vi "Refrigeration #2.vi"() -> ()   [LabVIEW 2017]
uses:
  Halt Refrig.vi
panel:
  out "Electric Motor Power":dbl caption="W" format="%.1f"
  out "Compressure Suction Pressure":dbl(knob)
  out "Compressor Discharge Pressure":dbl(knob) scale=0.0..60.0
  out "P2":dbl caption="psig" format="%.1g"
  out "P1":dbl caption="psig" format="%.1g"
  out "Evaporator Exit Temperature":dbl format="%.1g"
  out "Evaporator Entrance Temperature":dbl format="%.1g"
  out "Condensor Entrance Temperature":dbl format="%.1g"
  out "Condensor Exit Temperature":dbl format="%.1g"
  out "Compressor Exit Temperature":dbl format="%.1g"
  out "Compressor Entrance Temperature":dbl format="%.1g"
  out "Low Pressure Reciever Temperature":dbl format="%.1g"
  in  "stop":bool
  out "Data Point Count":i32
  in  "Specify Time between Data Points (sec)":dbl=1.0
  in  "Cancel Data Collection":bool
  in  "Specify number of data points":i16=1
  in  "Enable 3":bool
  out "Saving Data 3":bool
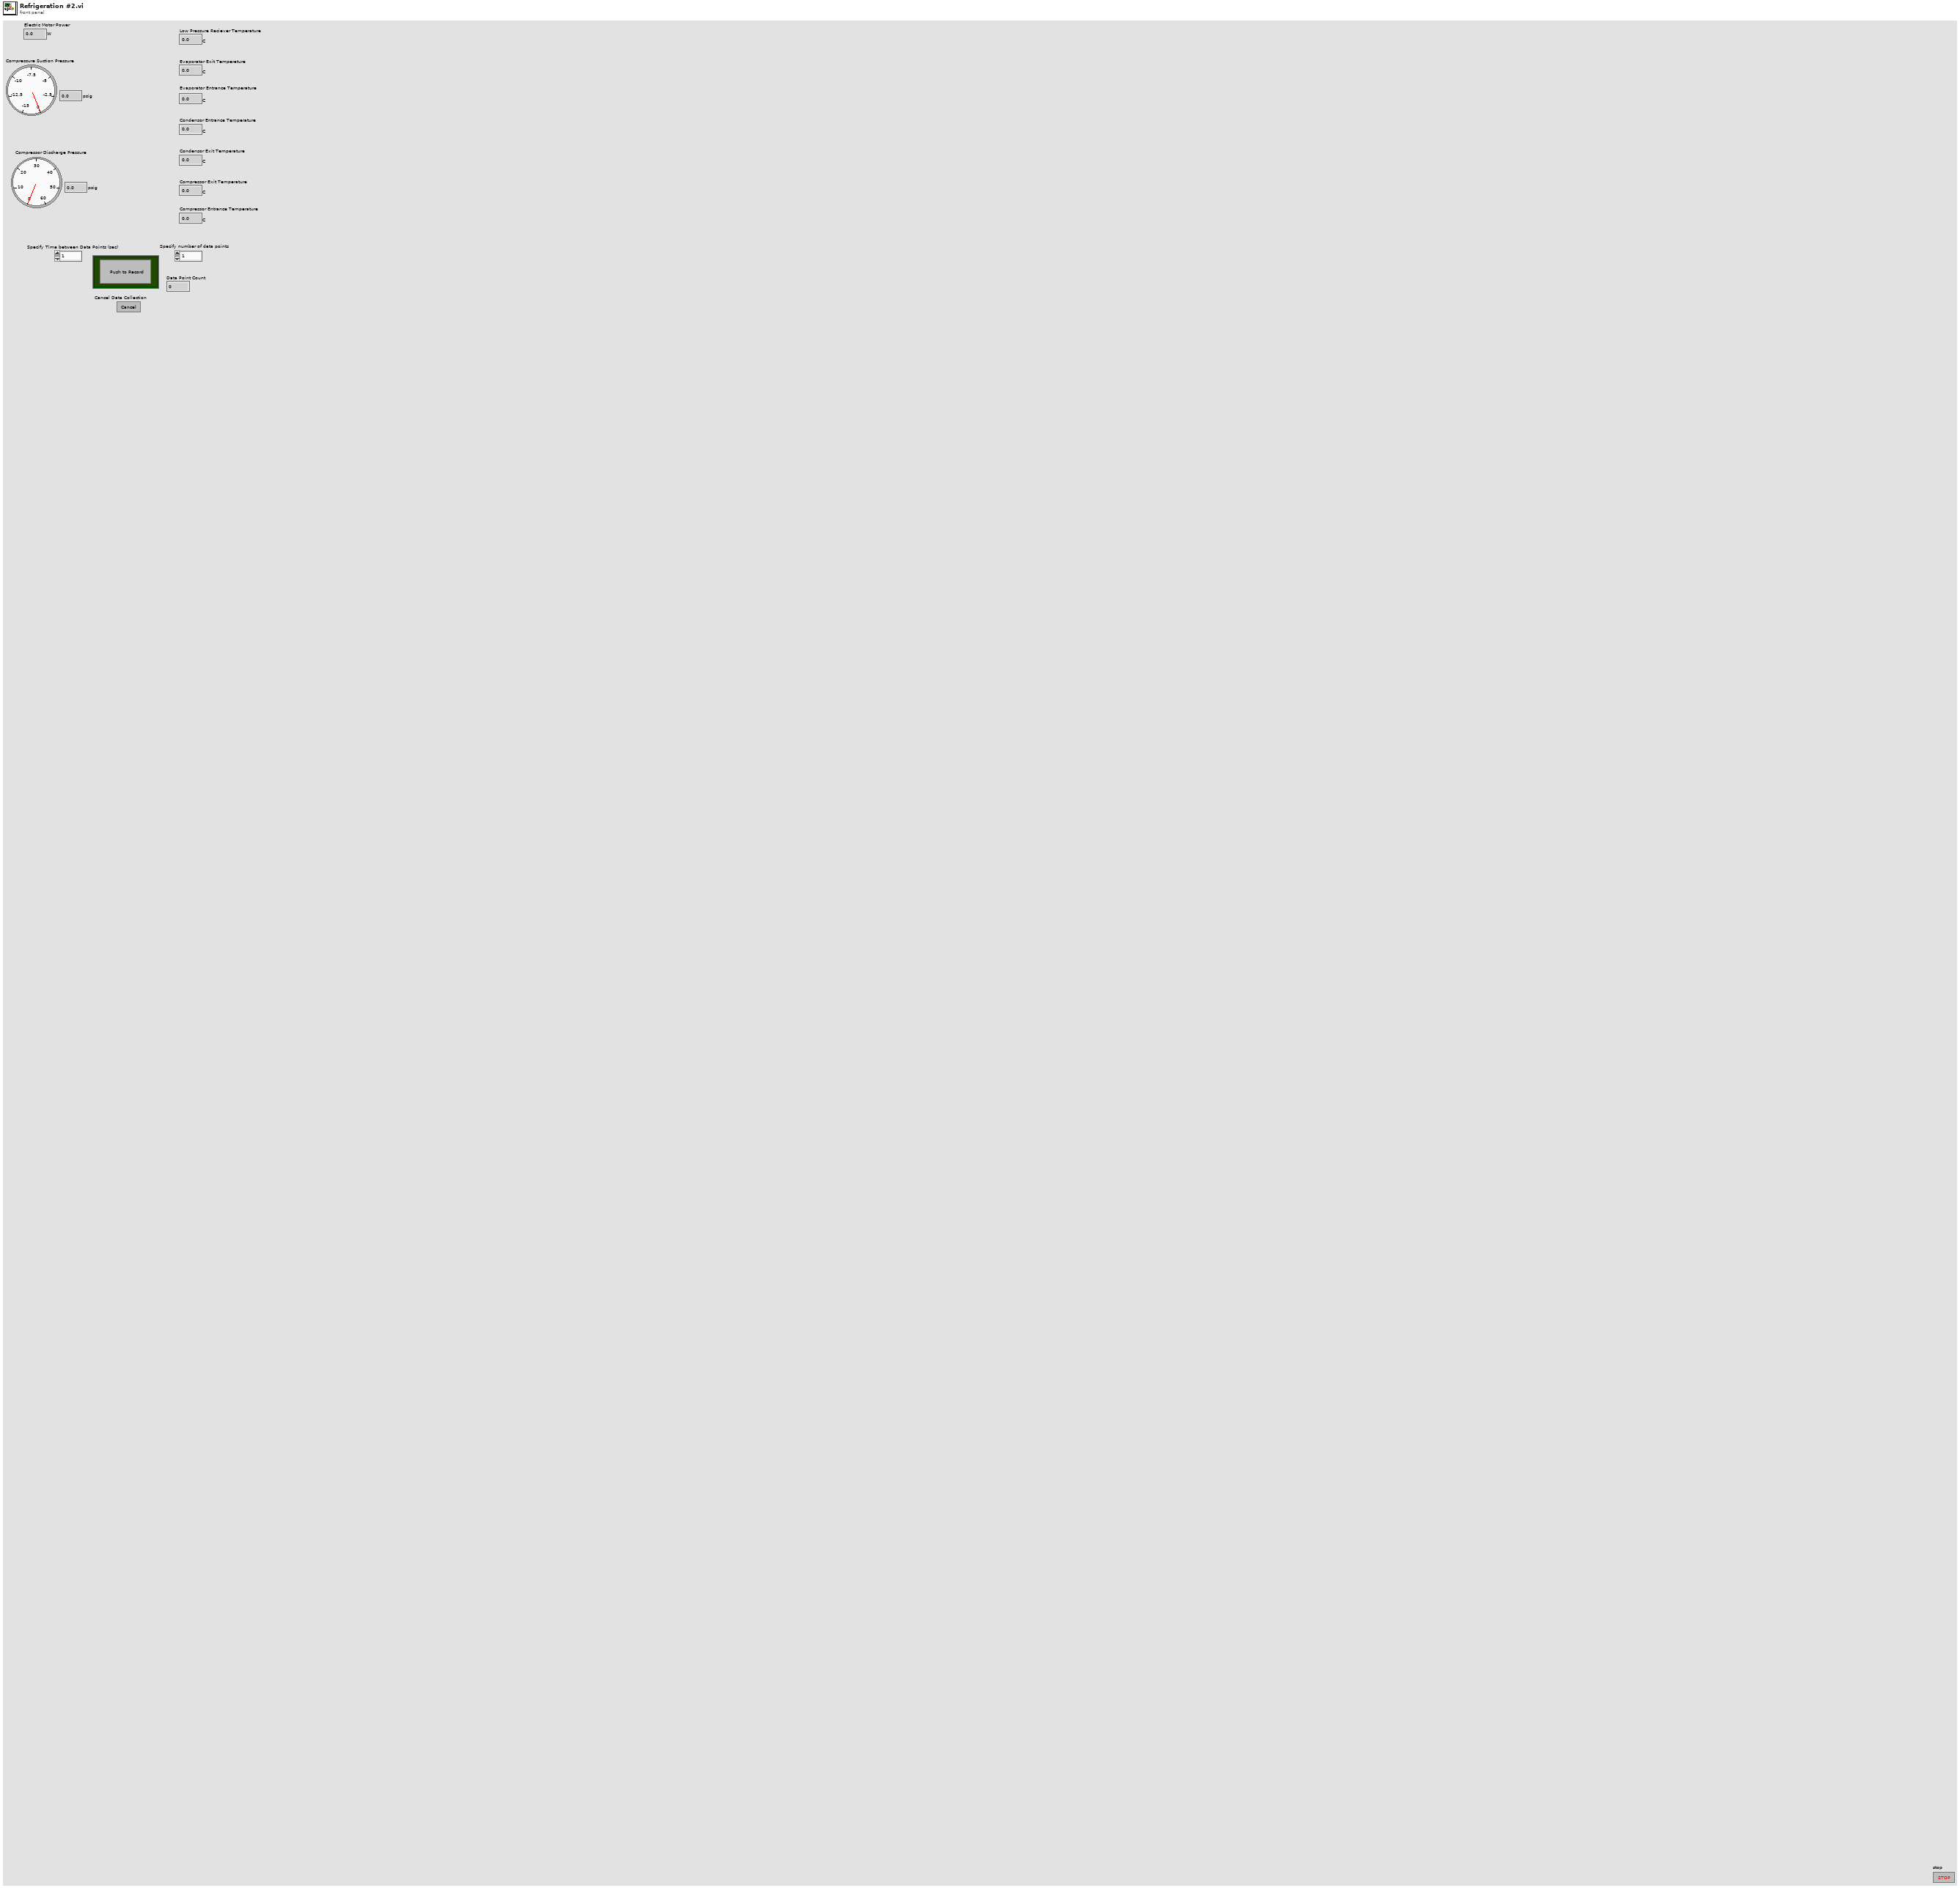
[diagram p1: front panel]
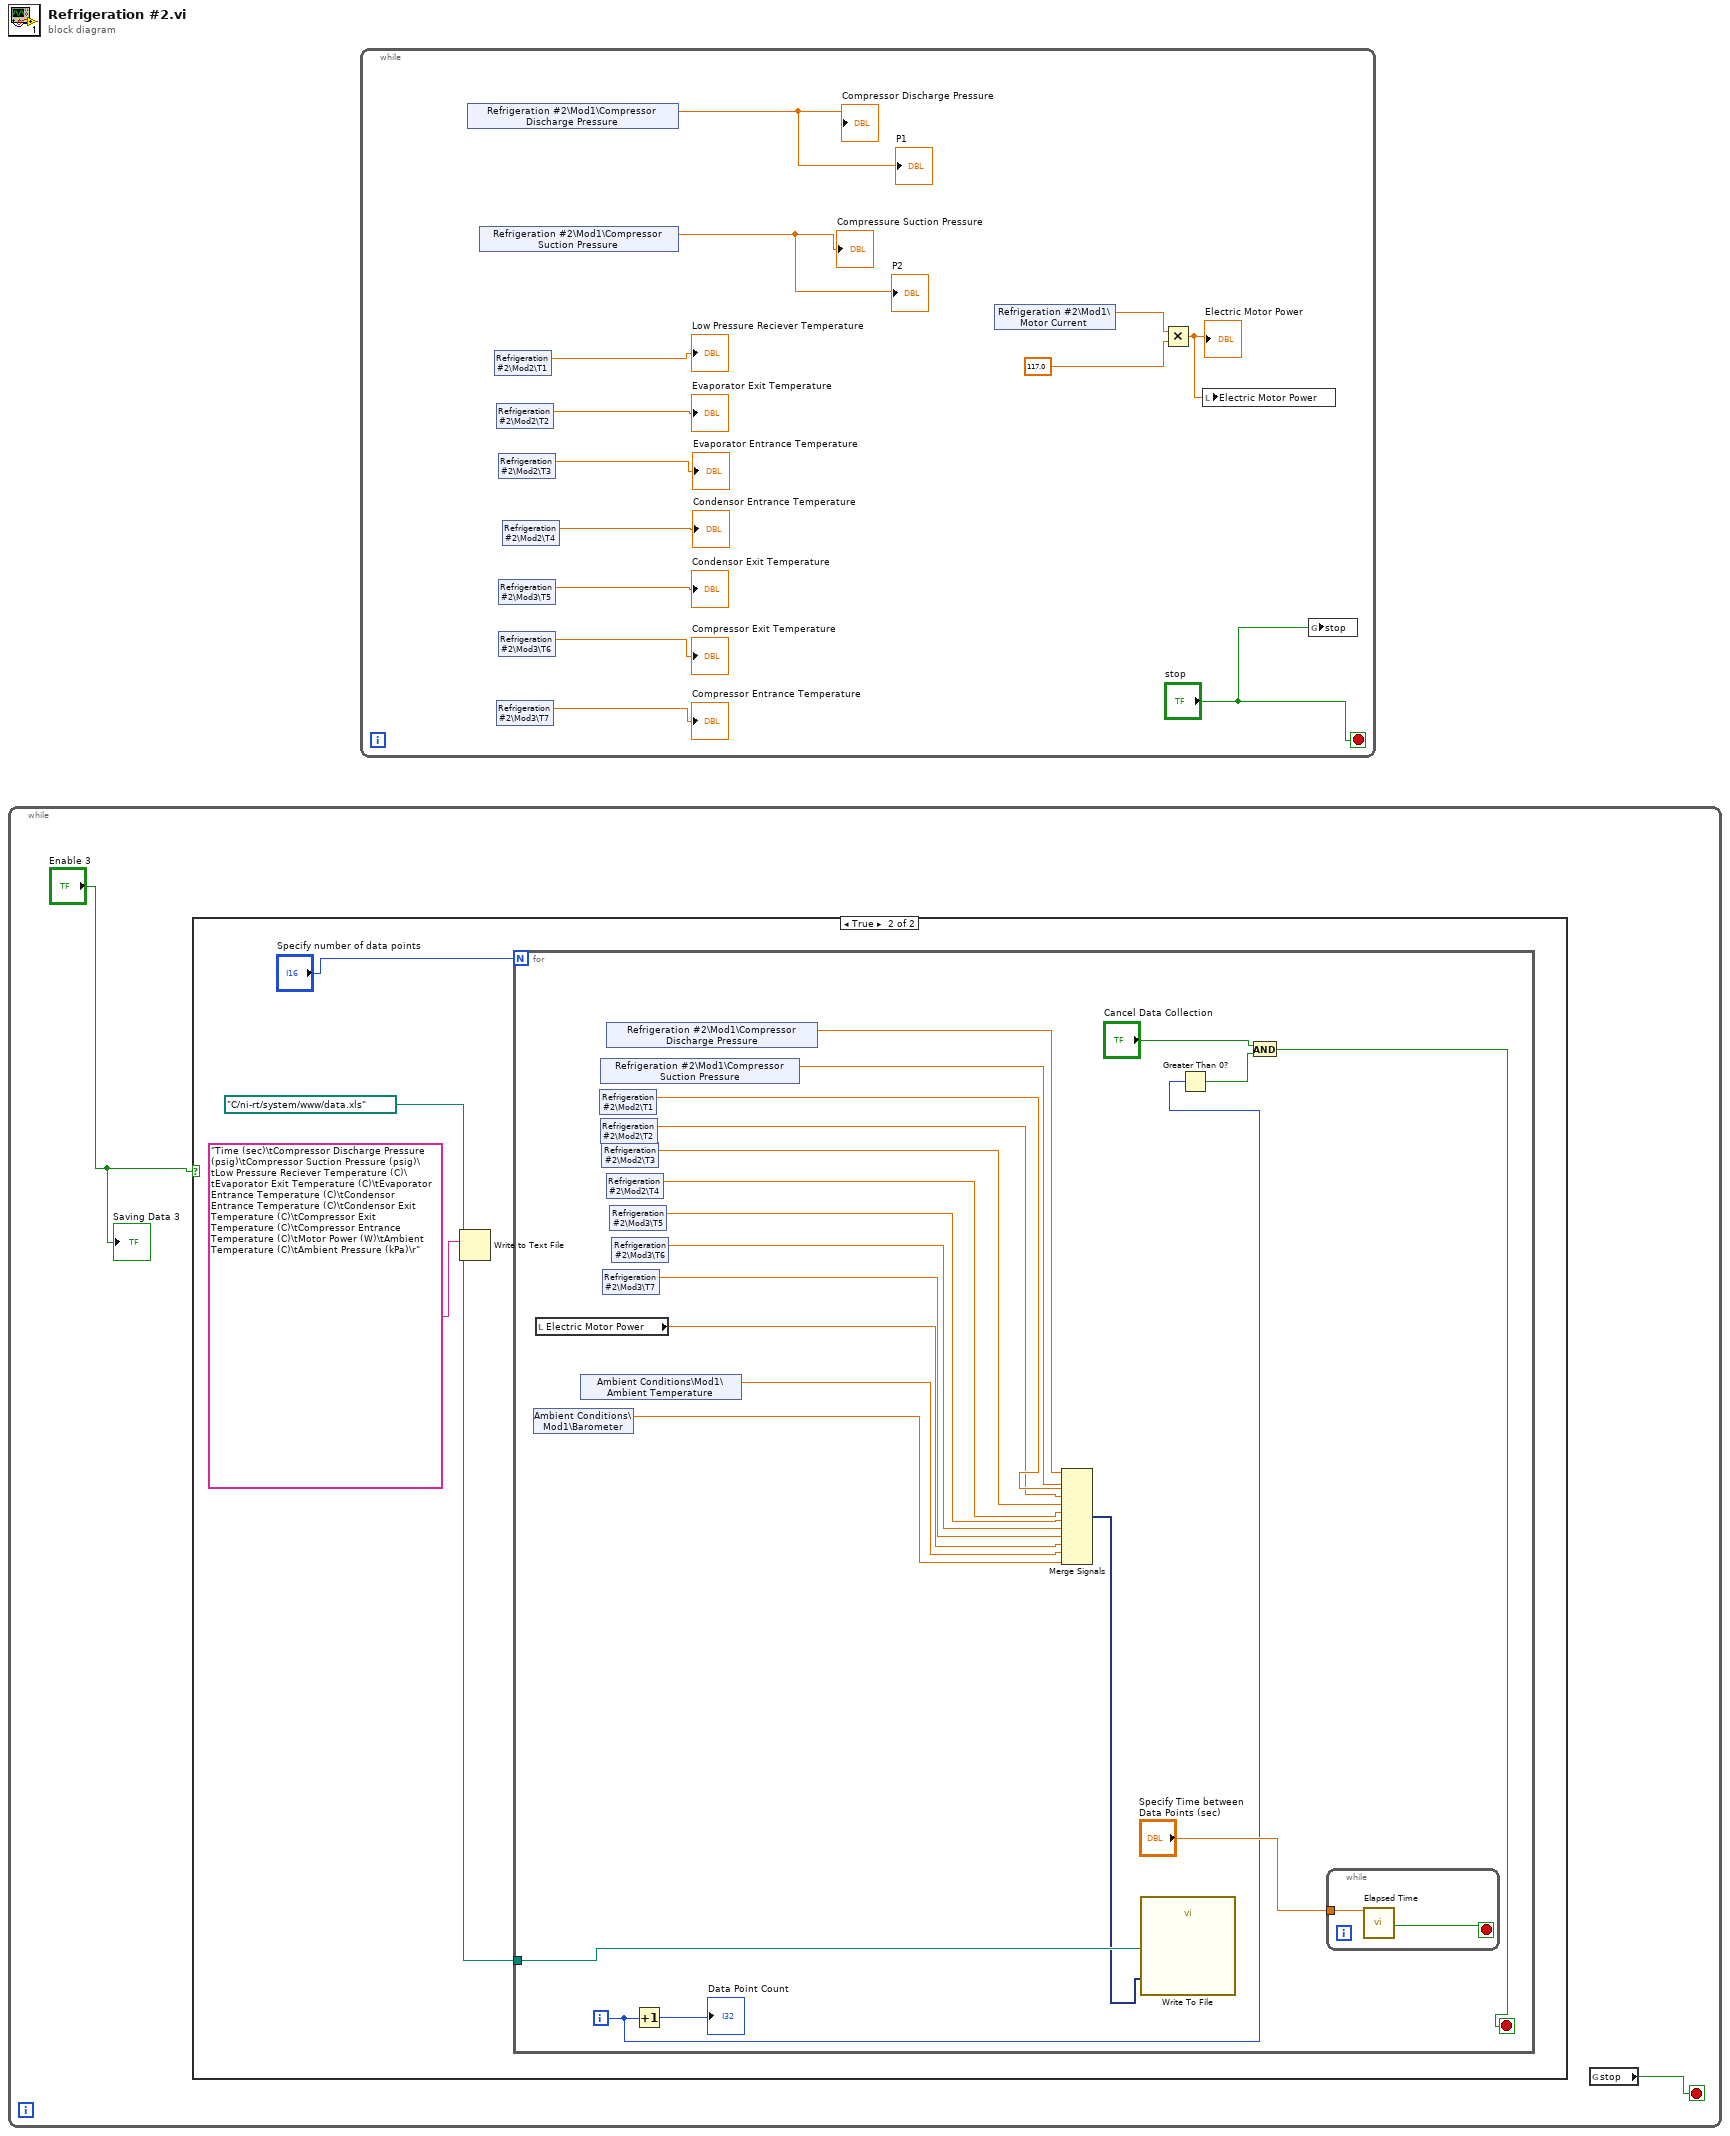
[diagram p0: block diagram]
diagram:
  n1 = while {
    stop <- w1 stop-if-true
    n2 = case shown="True" "Enable 3" {
      frame False {
      }
      frame True {
        w4 = path "C:/ni-rt/system/www/data.xls" ("Filename")
        n3 = Write to Text File(file (use dialog)=w4, text="Time (sec)\tCompressor Discharge Pressure (psig)\tCompressor Suction Pressure (psig)\tLow Pressure Reciever Temperature (C)\tEvaporator Exit Temperature (C)\tEvaporator Entrance Temperature (C)\tCondensor Entrance Temperature (C)\tCondensor Exit Temperature (C)\tCompressor Exit Temperature (C)\tCompressor Entrance Temperature (C)\tMotor Power (W)\tAmbient Temperature (C)\tAmbient Pressure (kPa)\r") -> ()  [unwired: 2 in, 3 out]
        n4 = for {
          N: "Specify number of data points" -> [_]
          tunnel: w4 -> [w25]
          i -> [w19]
          stop <- w16 stop-if-true
          n5 = shared-variable "Ambient Conditions\\Mod1\\Barometer"() -> (w8:dbl)  [unwired: 1 in, 1 out]
          n6 = local read "Electric Motor Power"() -> (w6:dbl)
          n7 = shared-variable "Ambient Conditions\\Mod1\\Ambient Temperature"() -> (w7:dbl)  [unwired: 1 in, 1 out]
          n8 = shared-variable "Refrigeration #2\\Mod2\\T1"() -> (w22:dbl)  [unwired: 1 in, 1 out]
          n9 = shared-variable "Refrigeration #2\\Mod1\\Compressor Suction Pressure"() -> (w23:dbl)  [unwired: 1 in, 1 out]
          n10 = shared-variable "Refrigeration #2\\Mod2\\T2"() -> (w15:dbl)  [unwired: 1 in, 1 out]
          n11 = shared-variable "Refrigeration #2\\Mod2\\T3"() -> (w14:dbl)  [unwired: 1 in, 1 out]
          n12 = shared-variable "Refrigeration #2\\Mod3\\T7"() -> (w9:dbl)  [unwired: 1 in, 1 out]
          n13 = shared-variable "Refrigeration #2\\Mod1\\Compressor Discharge Pressure"() -> (w11:dbl)  [unwired: 1 in, 1 out]
          n14 = shared-variable "Refrigeration #2\\Mod2\\T4"() -> (w13:dbl)  [unwired: 1 in, 1 out]
          n15 = shared-variable "Refrigeration #2\\Mod3\\T5"() -> (w12:dbl)  [unwired: 1 in, 1 out]
          n16 = shared-variable "Refrigeration #2\\Mod3\\T6"() -> (w10:dbl)  [unwired: 1 in, 1 out]
          n17 = Increment(x=w19) -> (x+1=→"Data Point Count":i32)
          n18 = Merge Signals(w11, w23, w22, w15, w14, w13, w12, w10, w9, w6, w7, w8) -> (w21:dynamicdata)
          n19 = call "Write To File"("Signals"=w21, "Filename"=w25) -> ()  [unwired: 15 in, 3 out]
          n20 = Greater Than 0?(x=w19) -> (x > 0?=w17:bool)
          n21 = And(x="Cancel Data Collection", y=w17) -> (x .and. y?=w16:bool)
          n22 = while {
            tunnel: "Specify Time between Data Points (sec)" -> [w26]
            stop <- w27 stop-if-true
            n23 = call "Elapsed Time"("Time Target (s)"=w26) -> ("Time has Elapsed"=w27:bool)  [unwired: 11 in, 7 out]
          }
        }
      }
    }
    n24 = global read "Halt Refrig.vi" "stop"() -> (w1:bool)
    "Saving Data 3" <- "Enable 3"
  }
  n25 = while {
    stop <- "stop" stop-if-true
    n26 = shared-variable "Refrigeration #2\\Mod1\\Compressor Discharge Pressure"() -> (→"Compressor Discharge Pressure" →"P1":dbl)  [unwired: 1 in, 1 out]
    n27 = shared-variable "Refrigeration #2\\Mod1\\Compressor Suction Pressure"() -> (→"Compressure Suction Pressure" →"P2":dbl)  [unwired: 1 in, 1 out]
    n28 = shared-variable "Refrigeration #2\\Mod2\\T1"() -> (→"Low Pressure Reciever Temperature":dbl)  [unwired: 1 in, 1 out]
    n29 = shared-variable "Refrigeration #2\\Mod2\\T2"() -> (→"Evaporator Exit Temperature":dbl)  [unwired: 1 in, 1 out]
    n30 = shared-variable "Refrigeration #2\\Mod3\\T7"() -> (→"Compressor Entrance Temperature":dbl)  [unwired: 1 in, 1 out]
    n31 = shared-variable "Refrigeration #2\\Mod2\\T3"() -> (→"Evaporator Entrance Temperature":dbl)  [unwired: 1 in, 1 out]
    n32 = shared-variable "Refrigeration #2\\Mod3\\T5"() -> (→"Condensor Exit Temperature":dbl)  [unwired: 1 in, 1 out]
    n33 = shared-variable "Refrigeration #2\\Mod3\\T6"() -> (→"Compressor Exit Temperature":dbl)  [unwired: 1 in, 1 out]
    n34 = shared-variable "Refrigeration #2\\Mod2\\T4"() -> (→"Condensor Entrance Temperature":dbl)  [unwired: 1 in, 1 out]
    n35 = shared-variable "Refrigeration #2\\Mod1\\Motor Current"() -> (w28:dbl)  [unwired: 1 in, 1 out]
    n36 = Multiply(x=w28, y=117.0) -> (x*y=w29:dbl)
    "Electric Motor Power" <- w29
    n37 = local write "Electric Motor Power"(w29) -> ()
    n38 = global write "Halt Refrig.vi" "stop"("stop") -> ()
  }
